vi "Temperature controlled LEDs.vi"() -> ()   [LabVIEW 2021]
doc: "Lights up different LEDs depending on the temperature sensed by the TMP36."
uses:
  <vilib>/MakerHub/LINX/Public/Peripherals/Digital/Digital Write 1 Chan.vi
  <vilib>/MakerHub/LINX/Public/Peripherals/Digital/Digital Write N Chans.vi
  <vilib>/MakerHub/LINX/Private/Local IO/LinxDigitalWrite.vi
  <vilib>/MakerHub/LINX/Public/Utilities/Check Channel.vi
  <vilib>/MakerHub/LINX/Public/Utilities/Open Serial.vi
  <vilib>/MakerHub/LINX/Public/Sensors/Temperature/TMP3x/TMP36.vi
  <vilib>/MakerHub/LINX/Private/Utilties/Generate Error.vi
  <vilib>/MakerHub/LINX/LMH-LINX.lvlib
  <vilib>/MakerHub/LINX/Public/Sensors/Temperature/TMP3x/TMP3x.lvlib
panel:
  out "Temp F":dbl
  out "Temp C":dbl
  in  "Stop":bool
  out "Loop Rate (Hz)":u32
  in  "Hot LED":u8=13
  in  "Room temperature LED":u8=13
  in  "Cold LED":u8=13
  in  "Analog Channel":u8
  in  "Serial Port":refnum<visa-resource-name>
  # "Set digital pins for LED"
  # "Blue is 20C or colder\nRoom temperature is between 21C and 24C\nRed is 24C and hotter"
  # "Select serial port for device and analog chanel for DHT36"
  # "Temperature in degree Fahrenheit and degree Celsius"
  # "Stop button and loop rate (Hz)"
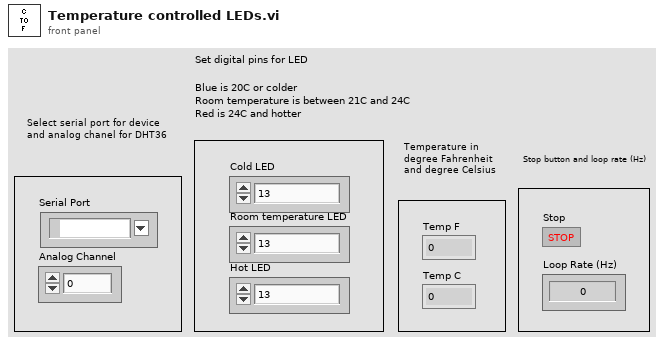
[diagram p1: front panel]
types:
  T1 = typedef "LMH-LINX.lvlib/LINX Ref.ctl" = cluster{"IO":T2, "Interface":T3, "LINX Device Config":T4}
  T2 = typedef "LMH-LINX.lvlib/Platform.ctl" = enum16{"Remote", "Local"}
  T3 = typedef "LMH-LINX.lvlib/Interface.ctl" = enum16{"Serial", "TCP"}
  T4 = typedef "LMH-LINX.lvlib/Device.lvlib/LINX Device Config.ctl" = cluster{"Interface":T3, "COM Port":refnum<visa-resource-name>, "TCP Configuration":T5, "Device Family":u8, "Device ID":u8, "Device Name":string, "TCP Ref":refnum<k5>, "Channels":T6}
  T5 = typedef "LMH-LINX.lvlib/Device.lvlib/TCP Config.ctl" = cluster{"IP Address":string, "Port":u16}
  T6 = typedef "LMH-LINX.lvlib/Channels.ctl" = cluster{"DI":u8[], "DO":u8[], "AI":u8[], "AO":u8[], "PWM":u8[], "QE":u8[], "UART":u8[], "I2C 2":u8[], "SPI":u8[], "CAN":u8[], "Servo":u8[], "AI Ref (V)":dbl, "AI Resolution (Bits)":u8, "AO Ref (V)":dbl, "AO Resolution (Bits)":u8}
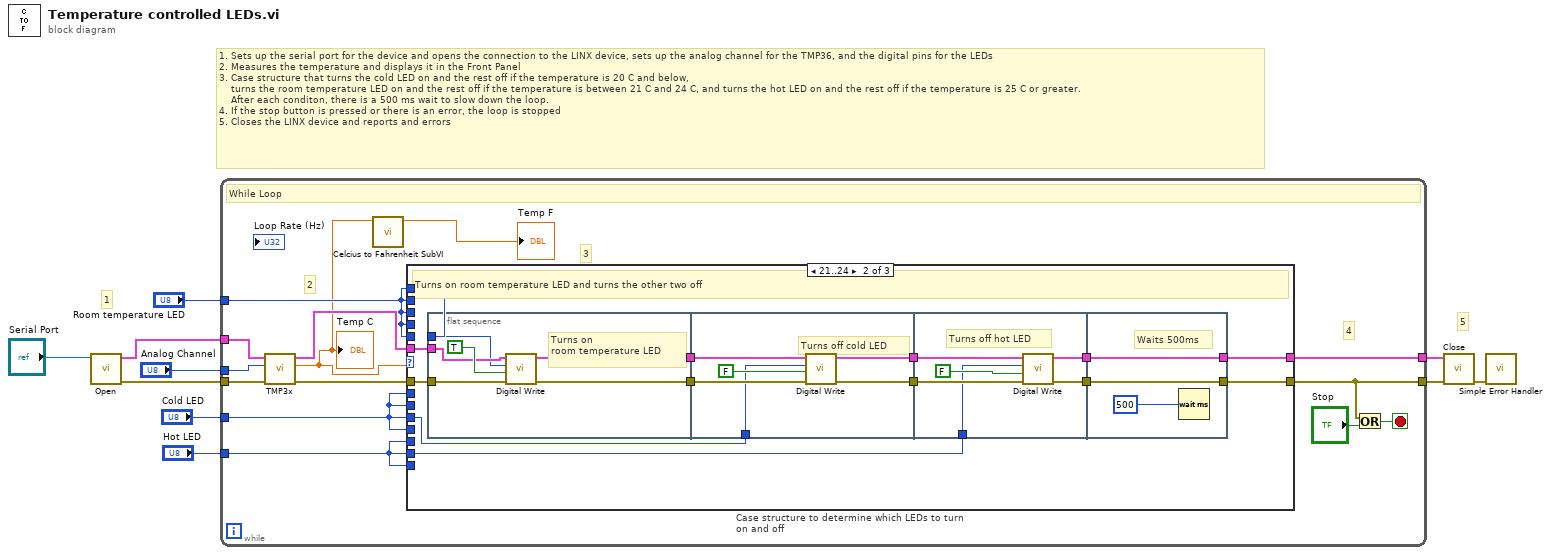
[diagram p0: block diagram]
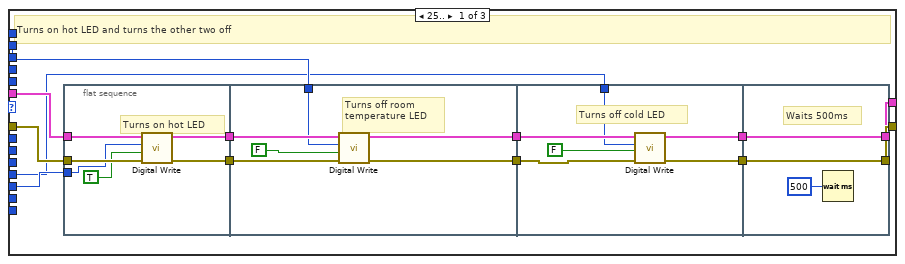
[diagram p2: hidden frame]
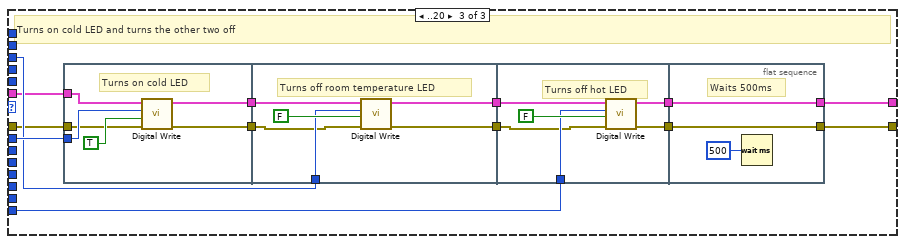
[diagram p3: hidden frame]
diagram:
  # "1. Sets up the serial port for the device and opens the connection to the LINX device, sets up the analog channel for the TMP36, and the digital pins for the LEDs\n2. Measures the temperature and displays it in the Front Panel\n3. Case structure that turns the cold LED on and the rest off if the temperature is 20 C and below, \n    turns the room temperature LED on and the rest off if the temperature is between 21 C and 24 C, and turns the hot LED on and the rest off if the temperature is 25 C or greater.\n    After each conditon, there is a 500 ms wait to slow down the loop.\n4. If the stop button is pressed or there is an error, the loop is stopped\n5. Closes the LINX device and reports and errors"
  # "5"
  # "1"
  n1 = call-poly <vilib>:"Open.vi"("Serial Port"="Serial Port") -> ("Error Out"=w8:errorcluster, "LINX Resource"=w9:T1)  [unwired: 8 in, 1 out]
  n2 = while {
    tunnel: w9 -> [w24]
    tunnel: w8 -> [w23]
    tunnel: "Analog Channel" -> [w22]
    tunnel: "Cold LED" -> [w15]
    tunnel: "Room temperature LED" -> [w14]
    tunnel: "Hot LED" -> [w13]
    tunnel: [w19] -> w2
    tunnel: [w18] -> w1
    stop <- w16 stop-if-true
    # "4"
    # "3"
    # "2"
    # "While Loop"
    n3 = call-poly <vilib>:"TMP3x.vi"("Error In"=w23, "Analog Channel"=w22, "LINX Resource"=w24) -> ("Error Out"=w20:errorcluster, "Temp C"=w12:dbl, "LINX Resource"=w21:T1)  [unwired: 6 in]
    "Temp C" <- w12
    n4 = call "Celcius to Fahrenheit SubVI.vi"("Temp C"=w12) -> ("Numeric"=→"Temp F":dbl)  [unwired: 10 in]
    n5 = case "Case structure to determine which LEDs to turn on and off" shown="21..24" w12 {
      tunnel: w21 -> [w35 w71 w102]
      tunnel: w20 -> [w37 w70 w96]
      tunnel: w15 -> [_ _ _]
      tunnel: w14 -> [_ _ _]
      tunnel: w13 -> [w36 _ _]
      tunnel: [w28 w62 w95] -> w19
      tunnel: [w29 w61 w97] -> w18
      tunnel: w14 -> [_ _ _]
      tunnel: w14 -> [w32 _ _]
      tunnel: w15 -> [w27 _ _]
      tunnel: w14 -> [_ w69 _]
      tunnel: w15 -> [_ w64 _]
      tunnel: w13 -> [_ w63 _]
      tunnel: w15 -> [_ _ w105]
      tunnel: w14 -> [_ _ w104]
      tunnel: w13 -> [_ _ w103]
      frame 25.. {
        # "Turns on hot LED and turns the other two off"
        n6 = flat-sequence {
          tunnel: w37 -> [w43]
          tunnel: w36 -> [w42]
          tunnel: w35 -> [w41]
          tunnel: [w39] -> w34
          tunnel: [w38] -> w33
          tunnel: w34 -> [w49]
          tunnel: w33 -> [w48]
          tunnel: w32 -> [w46]
          tunnel: [w45] -> w31
          tunnel: [w44] -> w30
          tunnel: w31 -> [w54]
          tunnel: w30 -> [w53]
          tunnel: w27 -> [w50]
          tunnel: [w52] -> w26
          tunnel: [w51] -> w25
          tunnel: [w57] -> w28
          tunnel: [w58] -> w29
          tunnel: w26 -> [w58]
          tunnel: w25 -> [w57]
          frame #0 {
            # "Turns on hot LED"
            n7 = call-poly <vilib>:"Digital Write.vi"("Error In"=w43, "Output Value"=TRUE, "DO Channel"=w42, "LINX Resource"=w41) -> ("Error Out"=w38:errorcluster, "LINX Resource"=w39:T1)  [unwired: 6 in]
          }
          frame #1 {
            # "Turns off room \ntemperature LED"
            n8 = call-poly <vilib>:"Digital Write.vi"("Error In"=w48, "Output Value"=FALSE, "DO Channel"=w46, "LINX Resource"=w49) -> ("Error Out"=w44:errorcluster, "LINX Resource"=w45:T1)  [unwired: 6 in]
          }
          frame #2 {
            # "Turns off cold LED"
            n9 = call-poly <vilib>:"Digital Write.vi"("Error In"=w53, "Output Value"=FALSE, "DO Channel"=w50, "LINX Resource"=w54) -> ("Error Out"=w52:errorcluster, "LINX Resource"=w51:T1)  [unwired: 6 in]
          }
          frame #3 {
            # "Waits 500ms"
            n10 = Wait (ms)(milliseconds to wait=500) -> ()  [unwired: 1 out]
          }
        }
      }
      frame 21..24 {
        # "Turns on room temperature LED and turns the other two off"
        n11 = flat-sequence {
          tunnel: w71 -> [w76]
          tunnel: w70 -> [w75]
          tunnel: w69 -> [w74]
          tunnel: [w73] -> w68
          tunnel: [w72] -> w67
          tunnel: w68 -> [w82]
          tunnel: w67 -> [w81]
          tunnel: [w80] -> w66
          tunnel: [w79] -> w65
          tunnel: w64 -> [w78]
          tunnel: w66 -> [w88]
          tunnel: w65 -> [w87]
          tunnel: w63 -> [w86]
          tunnel: [w85] -> w60
          tunnel: [w84] -> w59
          tunnel: [w91] -> w61
          tunnel: [w92] -> w62
          tunnel: w60 -> [w92]
          tunnel: w59 -> [w91]
          frame #0 {
            # "Turns on \nroom temperature LED"
            n12 = call-poly <vilib>:"Digital Write.vi"("Error In"=w75, "Output Value"=TRUE, "DO Channel"=w74, "LINX Resource"=w76) -> ("Error Out"=w72:errorcluster, "LINX Resource"=w73:T1)  [unwired: 6 in]
          }
          frame #1 {
            # "Turns off cold LED"
            n13 = call-poly <vilib>:"Digital Write.vi"("Error In"=w81, "Output Value"=FALSE, "DO Channel"=w78, "LINX Resource"=w82) -> ("Error Out"=w79:errorcluster, "LINX Resource"=w80:T1)  [unwired: 6 in]
          }
          frame #2 {
            # "Turns off hot LED"
            n14 = call-poly <vilib>:"Digital Write.vi"("Error In"=w87, "Output Value"=FALSE, "DO Channel"=w86, "LINX Resource"=w88) -> ("Error Out"=w84:errorcluster, "LINX Resource"=w85:T1)  [unwired: 6 in]
          }
          frame #3 {
            # "Waits 500ms"
            n15 = Wait (ms)(milliseconds to wait=500) -> ()  [unwired: 1 out]
          }
        }
      }
      frame ..20 {
        # "Turns on cold LED and turns the other two off"
        n16 = flat-sequence {
          tunnel: w105 -> [w110]
          tunnel: w102 -> [w109]
          tunnel: [w108] -> w101
          tunnel: [w107] -> w99
          tunnel: w96 -> [w106]
          tunnel: w104 -> [w116]
          tunnel: w101 -> [w115]
          tunnel: [w114] -> w100
          tunnel: w99 -> [w113]
          tunnel: [w112] -> w98
          tunnel: w103 -> [w122]
          tunnel: w100 -> [w121]
          tunnel: w98 -> [w120]
          tunnel: [w119] -> w94
          tunnel: [w118] -> w93
          tunnel: [w125] -> w95
          tunnel: [w126] -> w97
          tunnel: w94 -> [w126]
          tunnel: w93 -> [w125]
          frame #0 {
            # "Turns on cold LED"
            n17 = call-poly <vilib>:"Digital Write.vi"("Error In"=w106, "Output Value"=TRUE, "DO Channel"=w110, "LINX Resource"=w109) -> ("Error Out"=w107:errorcluster, "LINX Resource"=w108:T1)  [unwired: 6 in]
          }
          frame #1 {
            # "Turns off room temperature LED"
            n18 = call-poly <vilib>:"Digital Write.vi"("Error In"=w113, "Output Value"=FALSE, "DO Channel"=w116, "LINX Resource"=w115) -> ("Error Out"=w112:errorcluster, "LINX Resource"=w114:T1)  [unwired: 6 in]
          }
          frame #2 {
            # "Turns off hot LED"
            n19 = call-poly <vilib>:"Digital Write.vi"("Error In"=w120, "Output Value"=FALSE, "DO Channel"=w122, "LINX Resource"=w121) -> ("Error Out"=w119:errorcluster, "LINX Resource"=w118:T1)  [unwired: 6 in]
          }
          frame #3 {
            # "Waits 500ms"
            n20 = Wait (ms)(milliseconds to wait=500) -> ()  [unwired: 1 out]
          }
        }
      }
    }
    n21 = Or(x=w18, y="Stop") -> (x .or. y?=w16:bool)
  }
  n22 = call <vilib>:"Close.vi"("Error In"=w1, "LINX Resource"=w2) -> ("Error Out"=w3:errorcluster)  [unwired: 9 in]
  n23 = call <vilib>:"Simple Error Handler.vi"("error in (no error)"=w3) -> ()  [unwired: 4 in, 5 out]
